vi "n calculator.vi"(9 "yc":dbl, 10 "xc":dbl) -> (2 "n":dbl)   [LabVIEW 2014, in "AMS TS3472 Light Sensor.lvlib" / "AMS TCS3472.lvclass"]
uses:
  AMS TCS3472.lvclass
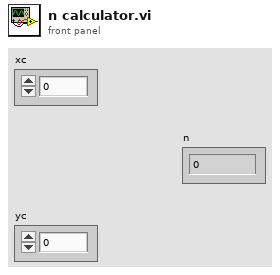
[diagram p1: front panel]
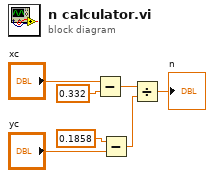
[diagram p0: block diagram]
diagram:
  n1 = Subtract(x="xc", y=0.332) -> (x-y=w3:dbl)
  n2 = Subtract(x=0.1858, y="yc") -> (x-y=w2:dbl)
  n3 = Divide(x=w3, y=w2) -> (x/y=→"n":dbl)
